vi "Get status bits 1 (G).vi"(0 "VISA resource name in":refnum<visa-resource-name>, 5 "Error In":errorcluster) -> (7 "nFaults":u8, 9 "nSensors":u8, 11 "nCards":u8, 13 "PowerState":bool, 14 "VISA resource name out":refnum<visa-resource-name>, 18 "ACK":bool, 19 "Error out":errorcluster)   [LabVIEW 2015]
uses:
  Ctls/Cmd str.ctl
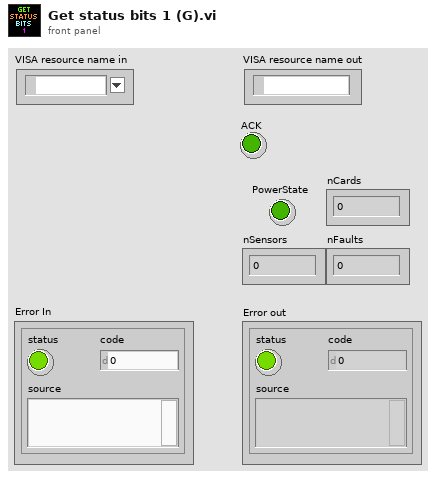
[diagram p1: front panel]
types:
  T1 = typedef "Cmd str.ctl" = string
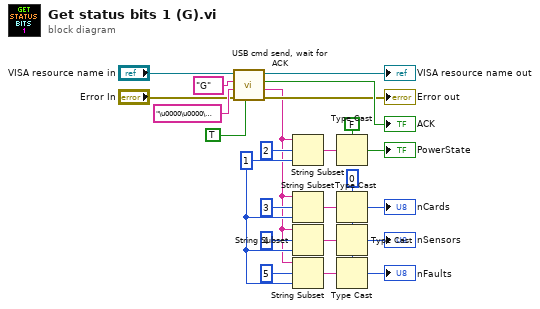
[diagram p0: block diagram]
diagram:
  w3 = u8 0 ("offset (0)")
  w12 = 1 ("length (rest)")
  n1 = call "USB cmd send, wait for ACK.vi"("Wait for ACK?"=TRUE, "Error In"="Error In", "4 byte config str"="\u0000\u0000\u0000\u0000", "Cmd"=T1 "G", "VISA resource name in"="VISA resource name in") -> ("Error out"=→"Error out":errorcluster, "Return msg"=w6:string, "ACK ok"=→"ACK":bool, "VISA resource name out"=→"VISA resource name out":refnum<visa-resource-name>)  [unwired: 1 in]
  n2 = String Subset(string=w6, offset (0)=2, length (rest)=w12) -> (substring=w11:string)
  n3 = String Subset(string=w6, offset (0)=3, length (rest)=w12) -> (substring=w10:string)
  n4 = String Subset(string=w6, offset (0)=4, length (rest)=w12) -> (substring=w9:string)
  n5 = String Subset(string=w6, offset (0)=5, length (rest)=w12) -> (substring=w8:string)
  n6 = Type Cast(type=FALSE, x=w11) -> (*(type *) &x=→"PowerState":bool)
  n7 = Type Cast(type=w3, x=w10) -> (*(type *) &x=→"nCards":u8)
  n8 = Type Cast(type=w3, x=w9) -> (*(type *) &x=→"nSensors":u8)
  n9 = Type Cast(type=w3, x=w8) -> (*(type *) &x=→"nFaults":u8)
